vi "CAPTH-Insert Data.vi"(0 "Runtime":T2, 5 "Threshold":dbl, 9 "stimcon":T1, 11 "error in (no error)":errorcluster, 12 "data":T3(array[cluster])) -> (8 "Plot Array":cluster{"Freq":dbl[], "Threshold":dbl[]}[](array[cluster]), 14 "data out":T3(array[cluster]), 15 "error out":errorcluster)   [LabVIEW 2020]
uses:
  Typedefs/CAPTH-Runtime.ctl
  Typedefs/CAPTH-StimCon.ctl
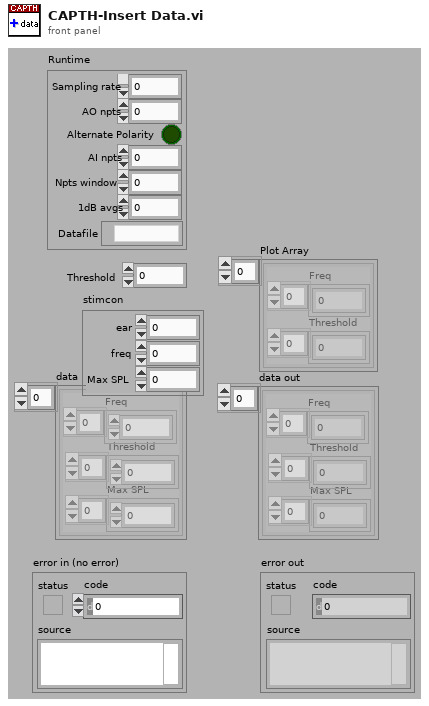
[diagram p1: front panel]
types:
  T1 = typedef "CAPTH-StimCon.ctl" = cluster{"ear":i32, "freq":i32, "Max SPL":dbl}
  T2 = typedef "CAPTH-Runtime.ctl" = cluster{"Sampling rate":dbl, "AO npts":i32, "Alternate Polarity":bool, "AI npts":i32, "Npts window":i32, "1dB avgs":i32, "Datafile":path}
  T3 = cluster{"Freq":dbl[], "Threshold":dbl[], "Max SPL":dbl[]}[]
  T4 = cluster{"Freq":dbl[], "Threshold":dbl[], "Max SPL":dbl[]}
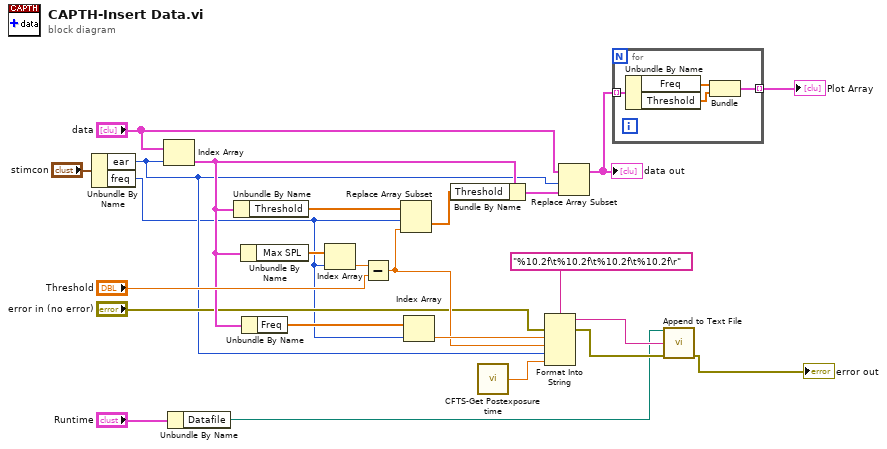
[diagram p0: block diagram]
diagram:
  n1 = Unbundle By Name("stimcon") -> ("ear"=w2:i32, "freq"=w1:i32)
  n2 = Index Array(array="data", index=w2) -> (element=w15:T4)
  n3 = Unbundle By Name("Runtime") -> ("Datafile"=w4:path)
  n4 = Unbundle By Name(w15) -> ("Threshold"=w24:dbl[])
  n5 = Unbundle By Name(w15) -> ("Max SPL"=w20:dbl[])
  n6 = Unbundle By Name(w15) -> ("Freq"=w14:dbl[])
  n7 = Index Array(array=w20, index=w1) -> (element=w19:dbl)
  n8 = Subtract(x=w19, y="Threshold") -> (x-y=w11:dbl)
  n9 = Replace Array Subset(array=w24, new element=w11, index=w1) -> (w23:dbl[])
  n10 = Index Array(array=w14, index=w1) -> (element=w12:dbl)
  n11 = Bundle By Name(cluster=w15, "Threshold"=w23) -> (w22:T4)
  n12 = call "CFTS-Get Postexposure time.vi"() -> ("Postexposure Time (min)"=w5:dbl)  [unwired: 14 in, 1 out]
  n13 = Format Into String(format string="%10.2f\t%10.2f\t%10.2f\t%10.2f\r", error in="error in (no error)", w12, w11, w2, w5) -> (resulting string=w9:string, error out=w7:errorcluster)  [unwired: 1 in]
  n14 = Replace Array Subset(array="data", new element=w22, index=w2) -> (w17:T3)
  "data out" <- w17
  n15 = for {
    tunnel: w17 -> [w28] mode=indexing
    tunnel: [w25] -> w16 mode=indexing
    n16 = Unbundle By Name(w28) -> ("Freq"=w27:dbl[], "Threshold"=w26:dbl[])
    n17 = Bundle("Freq"=w27, "Threshold"=w26) -> (w25:cluster{"Freq":dbl[], "Threshold":dbl[]})  [unwired: 1 in]
  }
  "Plot Array" <- w16
  n18 = call "Append to Text File.vi"("file path"=w4, "text"=w9, "error in (no error)"=w7) -> ("error out"=→"error out":errorcluster)  [unwired: 11 in, 1 out]
